vi "last project on 30-12.vi"() -> ()   [LabVIEW 2018]
uses:
  <vilib>/DAQmx/write.llb/DAQmx Write (Counter Frequency 1Chan 1Samp).vi
  <vilib>/DAQmx/write.llb/DAQmx Write (Digital 1D Bool NChan 1Samp 1Line).vi
  <vilib>/DAQmx/create/channels.llb/DAQmx Create Channel (DO-Digital Output).vi
  <vilib>/DAQmx/create/channels.llb/DAQmx Create Channel (CO-Pulse Generation-Frequency).vi
  <vilib>/DAQmx/configure/timing.llb/DAQmx Timing (Implicit).vi
  <vilib>/DAQmx/miscellaneous.llb/DAQmx Fill In Error Info.vi
panel:
  in  "Knob":dbl(knob) scale=0.0..1.0
  in  "frequency":dbl=1.0 format="%_6g"
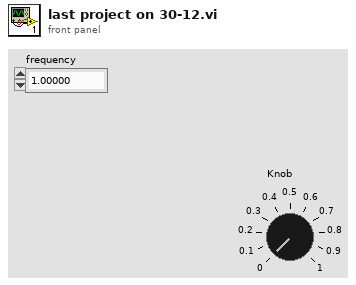
[diagram p1: front panel]
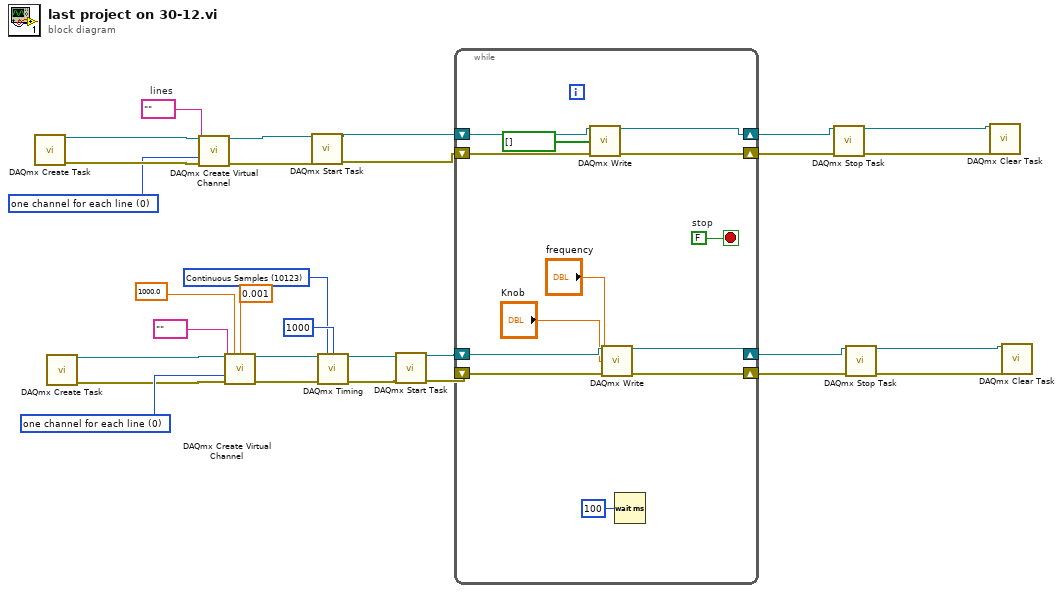
[diagram p0: block diagram]
diagram:
  w1 = 10123 items=["Finite Samples"=10178, "Continuous Samples"=10123, "Hardware Timed Single Point"=12522] ("sample mode")
  w15 = 0 items=["one channel for each line", "one channel for all lines"] ("line grouping")
  w21 = tag ""  # lines
  w22 = 0 items=["one channel for each line", "one channel for all lines"] ("line grouping")
  n1 = call <vilib>:"DAQmx Create Task.vi"() -> ("task out"=w26:refnum<k21>, "error out"=w25:errorcluster)  [unwired: 14 in]
  n2 = call <vilib>:"DAQmx Create Task.vi"() -> ("task out"=w13:refnum<k21>, "error out"=w14:errorcluster)  [unwired: 14 in]
  n3 = call-poly <vilib>:"DAQmx Create Virtual Channel.vi"("task in"=w26, "lines"=w21, "line grouping"=w22, "error in"=w25) -> ("task out"=w24:refnum<k21>, "error out"=w23:errorcluster)  [unwired: 10 in]
  n4 = call-poly <vilib>:"DAQmx Create Virtual Channel.vi"("task in"=w13, "frequency"=1000.0, "duty cycle"=0.001, "counter"=tag "" ("lines"), "units"=w15, "error in"=w14) -> ("task out"=w7:refnum<k21>, "error out"=w6:errorcluster)  [unwired: 8 in]
  n5 = call <vilib>:"DAQmx Start Task.vi"("task/channels in"=w24, "error in"=w23) -> ("task out"=w28:refnum<k21>, "error out"=w27:errorcluster)  [unwired: 12 in]
  n6 = call-poly <vilib>:"DAQmx Timing.vi"("task/channels in"=w7, "sample mode"=w1, "samples per channel"=1000, "error in"=w6) -> ("task out"=w5:refnum<k21>, "error out"=w4:errorcluster)  [unwired: 10 in]
  n7 = call <vilib>:"DAQmx Start Task.vi"("task/channels in"=w5, "error in"=w4) -> ("task out"=w3:refnum<k21>, "error out"=w12:errorcluster)  [unwired: 12 in]
  n8 = while {
    shift-right: [w41] -> w29
    shift-left: w27 -> [w40]
    shift-right: [w42] -> w30
    shift-left: w28 -> [w39]
    shift-right: [w37] -> w11
    shift-left: w12 -> [w38]
    shift-right: [w36] -> w10
    shift-left: w3 -> [w35]
    stop <- w31 stop-if-true
    w31 = FALSE  # stop
    n9 = call-poly <vilib>:"DAQmx Write.vi"("task/channels in"=w39, "data"=bool[] [], "error in"=w40) -> ("task out"=w42:refnum<k21>, "error out"=w41:errorcluster)  [unwired: 10 in, 1 out]
    n10 = call-poly <vilib>:"DAQmx Write.vi"("task/channels in"=w35, "frequency"="frequency", "duty cycle"="Knob", "error in"=w38) -> ("task out"=w36:refnum<k21>, "error out"=w37:errorcluster)  [unwired: 9 in, 1 out]
    n11 = Wait (ms)(milliseconds to wait=u32 100) -> ()  [unwired: 1 out]
  }
  n12 = call <vilib>:"DAQmx Stop Task.vi"("task/channels in"=w30, "error in"=w29) -> ("task out"=w20:refnum<k21>, "error out"=w19:errorcluster)  [unwired: 12 in]
  n13 = call <vilib>:"DAQmx Stop Task.vi"("task/channels in"=w10, "error in"=w11) -> ("task out"=w17:refnum<k21>, "error out"=w18:errorcluster)  [unwired: 12 in]
  n14 = call <vilib>:"DAQmx Clear Task.vi"("task in"=w20, "error in"=w19) -> ()  [unwired: 13 in, 1 out]
  n15 = call <vilib>:"DAQmx Clear Task.vi"("task in"=w17, "error in"=w18) -> ()  [unwired: 13 in, 1 out]
